vi "test Acyclic Loopback Multiple Pretrigger Writes.vi"(8 "error in":errorcluster, 11 "TestCase in":refnum<class "Octal Loopback.lvclass">) -> (0 "error out":errorcluster, 3 "TestCase out":refnum<class "Octal Loopback.lvclass">)   [LabVIEW 2020, in "Octal Loopback.lvclass"]
uses:
  Octal Loopback.lvclass
  C:/Program Files (x86)/National Instruments/LabVIEW 2020/vi.lib/NI/VeriStand Custom Device Testing Tools/VeriStandTestCase/VeriStandTestCase.lvclass
  <vilib>/numeric/Random Number (Range) U64.vi
  <vilib>/numeric/sub_Random U32.vi
  <vilib>/NI VeriStand/Execution/Workspace/NI VeriStand - Set Multiple Channel Values.vi
  <vilib>/addons/_JKI Toolkits/VI Tester/TestCase.llb/TestCase.lvclass
  <vilib>/NI VeriStand/Execution/Workspace/NI_VS Workspace ExecutionAPI.lvlib
  <vilib>/NI/VeriStand Custom Device Testing Tools/VeriStandTestUtilities/VeriStandTestUtilities.lvlib
  C:/Program Files (x86)/National Instruments/LabVIEW 2020/vi.lib/addons/_JKI Toolkits/VI Tester/TestCase.llb/TestCase.lvclass
  C:/Users/nitest/Desktop/Git 2020/niveristand-ballard-arinc429-custom-device/Source/Custom Device Support/Tests/System/Octal Loopback/Octal Loopback.lvclass
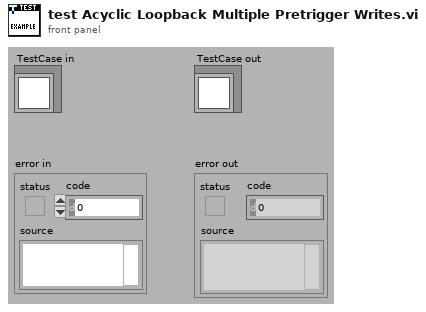
[diagram p1: front panel]
types:
  T1 = typedef "NI_VS Workspace ExecutionAPI.lvlib/WorkspaceAPI.ctl" = refnum<k24>
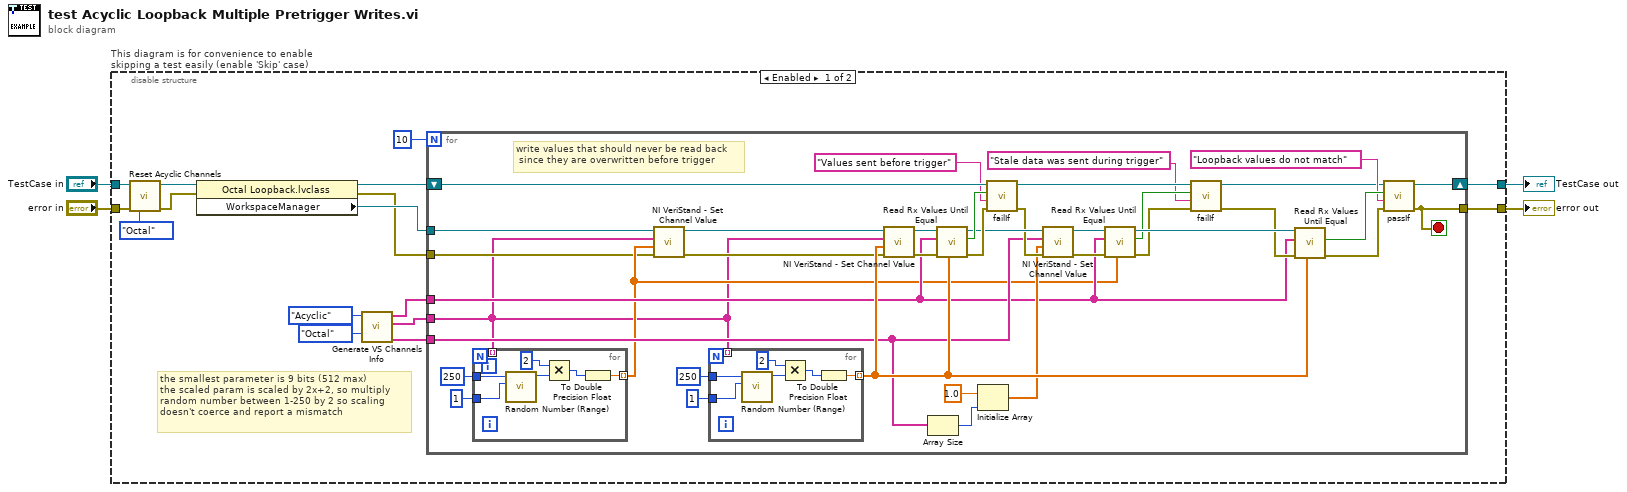
[diagram p0: block diagram]
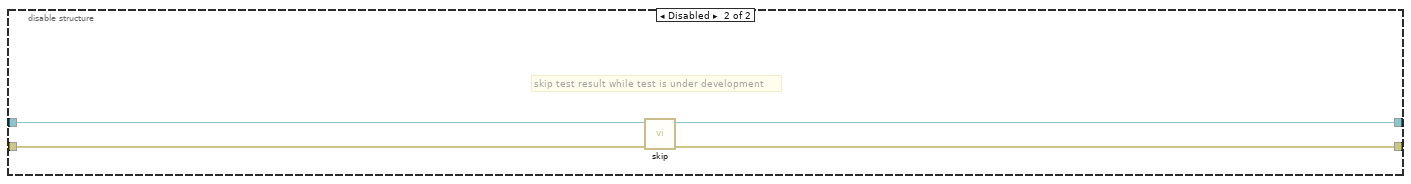
[diagram p2: hidden frame]
diagram:
  n1 = disable-structure "This diagram is for convenience to enable skipping a test easily (enable 'Skip' case)" shown="Enabled" {
    disable-tunnel: "TestCase in" -> [w7 w74]
    disable-tunnel: [w14 w72] -> w1
    disable-tunnel: [w13 w73] -> w3
    disable-tunnel: "error in" -> [w15 w71]
    frame Enabled {
      # "the smallest parameter is 9 bits (512 max)\nthe scaled param is scaled by 2x+2, so multiply \nrandom number between 1-250 by 2 so scaling\ndoesn't coerce and report a mismatch"
      n2 = call "Reset Acyclic Channels.vi"("error in (no error)"=w15, "Label Format (Decimal)"=enum16{"Decimal", "Octal"}."Octal", "reference in"=w7) -> ("error out"=w9:errorcluster, "reference out"=w8:refnum<class "Octal Loopback.lvclass">)  [unwired: 7 in]
      n3 = property class="Octal Loopback.lvclass"(reference=w8, error in=w9) -> (reference out=w17:refnum<class "Octal Loopback.lvclass">, error out=w18:errorcluster, "WorkspaceManager"=w19:T1)
      n4 = call "Generate VS Channels Info.vi"("Label Format (Decimal)"=enum16{"Decimal", "Octal"}."Octal", "Transfer Type"=enum16{"Acyclic", "Scheduled"}."Acyclic") -> ("Tx Trigger Channels Array"=w11:string[], "Tx Channels Array"=w12:string[], "Rx Channels Array"=w20:string[])  [unwired: 5 in, 2 out]
      n5 = for {
        N: 10 -> [_]
        tunnel: w20 -> [w28]
        tunnel: w19 -> [w25]
        tunnel: w18 -> [w22]
        tunnel: w12 -> [w21]
        shift-right: [w46] -> w14
        shift-left: w17 -> [w53]
        tunnel: [w45] -> w13
        tunnel: w11 -> [w40]
        stop <- w45 stop-if-true
        # "write values that should never be read back\n since they are overwritten before trigger"
        n6 = for {
          tunnel: [w63] -> w27 mode=indexing
          tunnel: u64 250 ("upper bound (100)") -> [w62]
          tunnel: u64 1 ("upper bound (100)") -> [w61]
          tunnel: w21 -> [_] mode=indexing
          n7 = call-poly <vilib>:"Random Number (Range).vi"("lower bound (0)"=w61, "upper bound (100)"=w62) -> ("number"=w64:u64)  [unwired: 9 in]
          n8 = Multiply(x=u64 2, y=w64) -> (x*y=w60:u64)
          n9 = To Double Precision Float(number=w60) -> (double precision float=w63:dbl)
        }
        n10 = call-poly <vilib>:"NI VeriStand - Set Channel Value.vi"("error in (no error)"=w22, "Values"=w27, "Channels"=w21, "WorkspaceManager in"=w25) -> ("error out"=w23:errorcluster, "WorkspaceManager out"=w24:T1)  [unwired: 6 in]
        n11 = for {
          tunnel: [w69] -> w49 mode=indexing
          tunnel: u64 250 ("upper bound (100)") -> [w68]
          tunnel: u64 1 ("upper bound (100)") -> [w67]
          tunnel: w21 -> [_] mode=indexing
          n12 = call-poly <vilib>:"Random Number (Range).vi"("lower bound (0)"=w67, "upper bound (100)"=w68) -> ("number"=w70:u64)  [unwired: 9 in]
          n13 = Multiply(x=u64 2, y=w70) -> (x*y=w66:u64)
          n14 = To Double Precision Float(number=w66) -> (double precision float=w69:dbl)
        }
        n15 = call-poly <vilib>:"NI VeriStand - Set Channel Value.vi"("error in (no error)"=w23, "Values"=w49, "Channels"=w21, "WorkspaceManager in"=w24) -> ("error out"=w54:errorcluster, "WorkspaceManager out"=w56:T1)  [unwired: 6 in]
        n16 = Array Size(array=w40) -> (size(s)=w39:i32)
        n17 = call <vilib>:"Read Rx Values Until Equal.vi"("expected values"=w49, "error in"=w54, "Rx aliases"=w28, "workspace manager in"=w56) -> ("error out"=w55:errorcluster, "values equal expected"=w52:bool, "workspace manager out"=w51:T1)  [unwired: 5 in]
        n18 = Initialize Array(1.0, w39) -> (w41:dbl[])
        n19 = call-dynamic "failIf.vi"("error in (no error)"=w55, "message (\"\")"="Values sent before trigger" ("message (\"\")"), "fail"=w52, "TestCase in"=w53) -> ("error out"=w50:errorcluster, "TestCase out"=w33:refnum<class "Octal Loopback.lvclass">)  [unwired: 6 in]
        n20 = call-poly <vilib>:"NI VeriStand - Set Channel Value.vi"("error in (no error)"=w50, "Values"=w41, "Channels"=w40, "WorkspaceManager in"=w51) -> ("error out"=w36:errorcluster, "WorkspaceManager out"=w35:T1)  [unwired: 6 in]
        n21 = call <vilib>:"Read Rx Values Until Equal.vi"("expected values"=w27, "error in"=w36, "Rx aliases"=w28, "workspace manager in"=w35) -> ("error out"=w31:errorcluster, "values equal expected"=w29:bool, "workspace manager out"=w34:T1)  [unwired: 5 in]
        n22 = call-dynamic "failIf.vi"("error in (no error)"=w31, "message (\"\")"="Stale data was sent during trigger" ("message (\"\")"), "fail"=w29, "TestCase in"=w33) -> ("error out"=w30:errorcluster, "TestCase out"=w32:refnum<class "Octal Loopback.lvclass">)  [unwired: 6 in]
        n23 = call <vilib>:"Read Rx Values Until Equal.vi"("expected values"=w49, "error in"=w30, "Rx aliases"=w28, "workspace manager in"=w34) -> ("error out"=w47:errorcluster, "values equal expected"=w48:bool)  [unwired: 5 in, 1 out]
        n24 = call-dynamic "passIf.vi"("error in (no error)"=w47, "message (\"\")"="Loopback values do not match" ("message (\"\")"), "pass"=w48, "TestCase in"=w32) -> ("error out"=w45:errorcluster, "TestCase out"=w46:refnum<class "Octal Loopback.lvclass">)  [unwired: 6 in]
      }
    }
    frame Disabled {
      # "skip test result while test is under development"
      n25 = call <vilib>:"skip.vi"("error in (no error)"=w71, "TestCase in"=w74) -> ("error out"=w73:errorcluster, "TestCase out"=w72:refnum<class "Octal Loopback.lvclass">)  [unwired: 8 in]
    }
  }
  "error out" <- w3
  "TestCase out" <- w1
